vi "Update Gains PID.vi"(0 "Error, e":dbl, 1 "Gains, Kp":dbl[](array[numeric]) format="%.3f", 2 "Update rate, mK":dbl[](array[numeric]) format="%.2e", 3 "Gamma, G":dbl, 4 "Tracking errors, e":dbl[](array[numeric]) format="%.3f") -> (5 "New gains, Kp":dbl[](array[numeric]) format="%.3f")   [LabVIEW 2022 SP3]
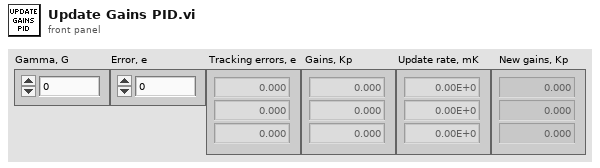
[diagram p1: front panel]
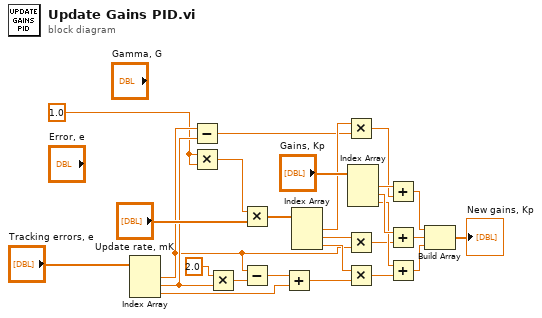
[diagram p0: block diagram]
diagram:
  w1 = 1.0
  n1 = Index Array(array="Tracking errors, e") -> (element #1=w13:dbl, element #2=w21:dbl, element #3=w18:dbl)  [unwired: 3 in]
  n2 = Subtract(x=w13, y=w21) -> (x-y=w14:dbl)
  n3 = Multiply(x=w1, y=w1) -> (x*y=w23:dbl)
  n4 = Multiply(x=2.0, y=w21) -> (x*y=w20:dbl)
  n5 = Multiply(x=w23, y="Update rate, mK") -> (x*y=w24:dbl[])
  n6 = Subtract(x=w13, y=w20) -> (x-y=w19:dbl)
  n7 = Add(x=w19, y=w18) -> (x+y=w12:dbl)
  n8 = Index Array(array=w24) -> (element #1=w17:dbl, element #2=w16:dbl, element #3=w15:dbl)  [unwired: 3 in]
  n9 = Multiply(x=w17, y=w14) -> (x*y=w8:dbl)
  n10 = Multiply(x=w16, y=w13) -> (x*y=w7:dbl)
  n11 = Multiply(x=w15, y=w12) -> (x*y=w6:dbl)
  n12 = Index Array(array="Gains, Kp") -> (element #1=w11:dbl, element #2=w10:dbl, element #3=w9:dbl)  [unwired: 3 in]
  n13 = Add(x=w11, y=w8) -> (x+y=w5:dbl)
  n14 = Add(x=w10, y=w7) -> (x+y=w4:dbl)
  n15 = Add(x=w9, y=w6) -> (x+y=w3:dbl)
  n16 = Build Array(w5, w4, w3) -> (→"New gains, Kp":dbl[])
